vi "单个流程校验.vi"(5 "简易流程Id":u16(ring), 6 "是否是简易流程":bool, 7 "添加的路径":path, 8 "error in (no error)":errorcluster caption="错误输入（无错误）", 9 "量程":enum16{"低量程", "高量程"}(ring), 10 "测量模式":T1(ring), 11 "测量参数":u16(ring) items=["总氮"=2, "总磷"=1, "氨氮"=3, "COD"=22]) -> (0 "error out":errorcluster caption="错误输出", 2 "结果字符串":string, 3 "check？":bool)   [LabVIEW 2016, in "斯坦道总磷.lvlib"]
uses:
  <vilib>/Plasmionique/MB Master/MB Master.lvlib
panel:
  out "数组":u16[](array[numeric])
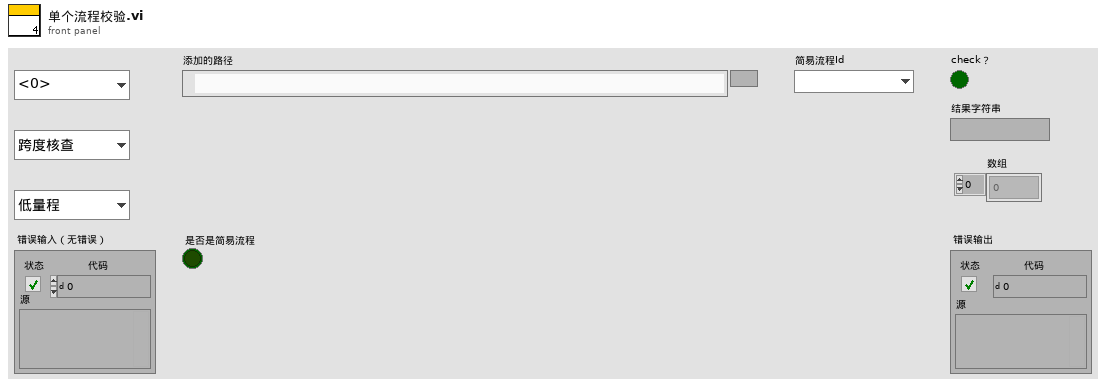
[diagram p1: front panel]
types:
  T1 = enum16{"跨度核查", "水样测量", "零点核查", "标样核查", "加标回收", "快捷测试", "空白校准", "标样校准"}
  T2 = cluster{"测量参数":u16, "测量模式":enum16{"跨度核查", "水样测量", "零点核查", "标样核查", "加标回收", "快捷测试", "空白校准", "标样校准"}, "量程":enum16{"低量程", "高量程"}}
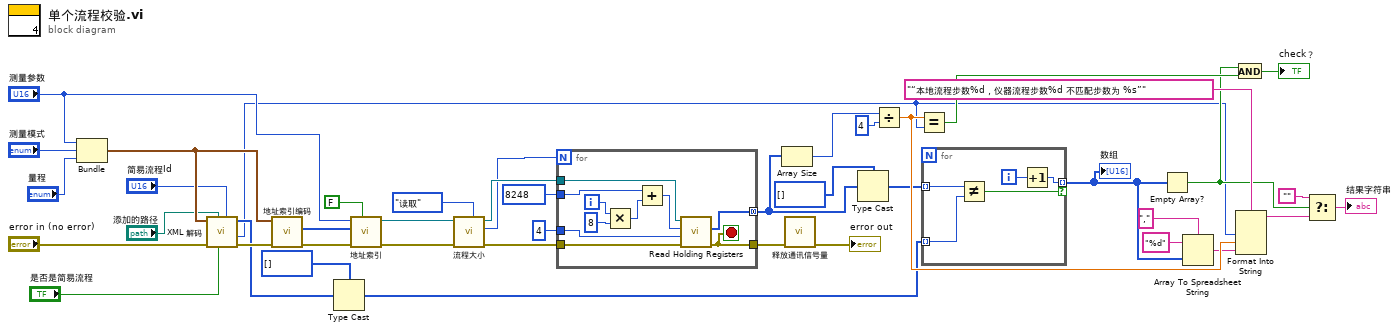
[diagram p0: block diagram]
diagram:
  n1 = Bundle("测量参数"="测量参数", "测量模式"="测量模式", "量程"="量程") -> (w10:T2)  [unwired: 1 in]
  n2 = call "XML 解码.vi"("简易流程Id"="简易流程Id", "是否是简易流程"="是否是简易流程", "添加的路径"="添加的路径", "error in (no error)"="error in (no error)", "参数簇"=w10) -> ("error out"=w9:errorcluster, "大小"=w1:i32, "步骤详情"=w2:u16[])  [unwired: 3 in, 1 out]
  n3 = call "地址索引编码.vi"("error in (no error)"=w9, "参数簇"=w10) -> ("error out"=w7:errorcluster, "数组"=w8:u16[])  [unwired: 8 in]
  n4 = Type Cast(type=u64[] [], x=w2) -> (*(type *) &x=w18:u64[])
  n5 = call "地址索引.vi"("4.2写公式？"=FALSE ("写流程？"), "error in (no error)"=w7, "values"=w8, "测量参数"="测量参数") -> ("error out"=w40:errorcluster, "MB session out"=w39:refnum<class "MB_Master.lvclass">)  [unwired: 6 in]
  n6 = call "流程大小.vi"("功能"=enum16{"写入", "读取"}."读取", "error in (no error)"=w40, "MB session in"=w39) -> ("error out"=w37:errorcluster, "大小读取"=w27:i32, "MB session out"=w38:refnum<class "MB_Master.lvclass">)  [unwired: 6 in]
  n7 = for {
    N: w27 -> [_]
    tunnel: u16 8248 ("starting address") -> [w53]
    tunnel: [w46] -> w36
    tunnel: w38 -> [w49]
    tunnel: w37 -> [w48]
    tunnel: [w45] -> w15 mode=concatenating
    tunnel: 4 ("y") -> [w44]
    i -> [w50]
    stop <- w46 stop-if-true
    n8 = Multiply(x=w50, y=8) -> (x*y=w52:i32)
    n9 = Add(x=w53, y=w52) -> (x+y=w47:i32)
    n10 = call <vilib>:"Read Holding Registers.vi"("error in (no error)"=w48, "quantity"=w44, "starting address"=w47, "MB session in"=w49) -> ("error out"=w46:errorcluster, "Registers"=w45:u16[])  [unwired: 5 in, 1 out]
  }
  n11 = Array Size(array=w15) -> (size(s)=w25:i32)
  n12 = call "释放通讯信号量.vi"("error in (no error)"=w36) -> ("error out"=→"error out":errorcluster)  [unwired: 10 in]
  n13 = Type Cast(type=u64[] [], x=w15) -> (*(type *) &x=w16:u64[])
  n14 = Divide(x=w25, y=4) -> (x/y=w26:dbl)
  n15 = Equal?(x=w26, y=w1) -> (x = y?=w33:bool)
  n16 = for {
    tunnel: w16 -> [w57] mode=indexing
    tunnel: w18 -> [w58] mode=indexing
    tunnel: [w54] -> w13 mode=indexing if=w56
    i -> [w55]
    n17 = Not Equal?(x=w57, y=w58) -> (x != y?=w56:bool)
    n18 = Increment(x=w55) -> (x+1=w54:i32)
  }
  "数组" <- w13
  n19 = Empty Array?(array=w13) -> (empty?=w22:bool)
  n20 = Array To Spreadsheet String(delimiter (Tab)="," ("分隔符(Tab)"), array=w13, 3:"%d" ("格式字符串")) -> (spreadsheet string=w23:string)
  n21 = And(x=w22, y=w33) -> (x .and. y?=→"check？":bool)
  n22 = Format Into String(format string="“本地流程步数%d，仪器流程步数%d 不匹配步数为 %s”" ("格式字符串"), w1, w26, w23) -> (resulting string=w21:string)  [unwired: 2 in, 1 out]
  n23 = Select(t="", s=w22, f=w21) -> (s? t:f=→"结果字符串":string)
